vi "testing.vi"() -> ()   [LabVIEW 2022 SP3]
uses:
  <vilib>/Instr/_visa.llb/VISA Configure Serial Port (Instr).vi
panel:
  out "unsigned byte array":dbl[](array[numeric])
  out "String":string
  in  "stop":bool
  in  "VISA resource name":refnum<visa-resource-name>
  in  "Connect":bool
  in  "Baudrate":string(combo)
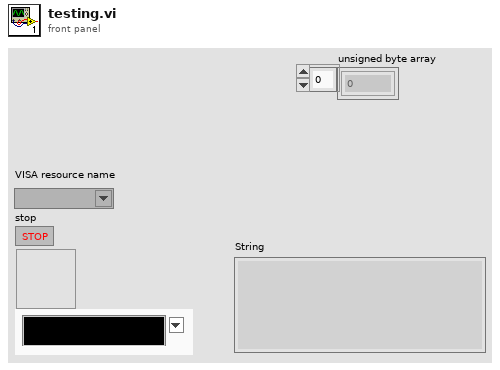
[diagram p1: front panel]
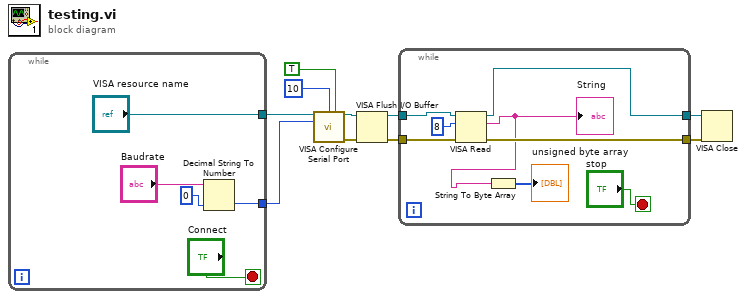
[diagram p0: block diagram]
diagram:
  n1 = while {
    tunnel: ["VISA resource name"] -> w7
    tunnel: [w14] -> w8
    stop <- "Connect" stop-if-true
    n2 = Decimal String To Number(string="Baudrate", default (0L)=0 ("default (0 I32)")) -> (number=w14:i32)  [unwired: 1 in, 1 out]
  }
  n3 = call-poly "VISA Configure Serial Port"("VISA resource name"=w7, "termination char\n(0xA = '\\n' = LF)"=u8 10 ("termination char\n(0xA = '\\n' = LF)"), "Enable Termination\nChar (T)"=TRUE ("Enable Termination\nChar (T)"), "baud rate (9600)"=w8) -> ("VISA resource name out"=w6:refnum<visa-resource-name>, "error out"=w5:errorcluster)  [unwired: 10 in]
  n4 = VISA Flush I/O Buffer(VISA resource name=w6, error in (no error)=w5) -> (VISA resource name out=w4:refnum<visa-resource-name>, error out=w3:errorcluster)  [unwired: 1 in]
  n5 = while {
    tunnel: w4 -> [w23]
    tunnel: w3 -> [w22]
    tunnel: [w20] -> w1
    tunnel: [w18] -> w2
    stop <- "stop" stop-if-true
    n6 = VISA Read(VISA resource name=w23, byte count=u32 8, error in (no error)=w22) -> (VISA resource name out=w20:refnum<visa-resource-name>, read buffer=w17:string, error out=w18:errorcluster)  [unwired: 1 out]
    "String" <- w17
    n7 = String To Byte Array(string=w17) -> (unsigned byte array=→"unsigned byte array":u8[])
  }
  n8 = VISA Close(VISA resource name=w1, error in (no error)=w2) -> ()  [unwired: 1 out]
